vi "Aircraft 8 RC Values .vi"(7 "Method":enum16{"Get", "Set"}(ring), 11 "Aircraft RC Data":T1) -> (3 "Aircraft RC Data 2":T1)   [LabVIEW 2014]
uses:
  Controls/Aircraft RC Data.ctl
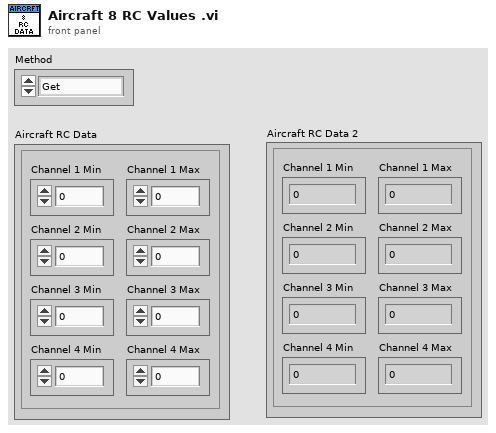
[diagram p1: front panel]
types:
  T1 = typedef "Aircraft RC Data.ctl" = cluster{"Channel 1 Min":i16, "Channel 1 Max":i16, "Channel 2 Min":i16, "Channel 2 Max":i16, "Channel 3 Min":i16, "Channel 3 Max":i16, "Channel 4 Min":i16, "Channel 4 Max":i16}
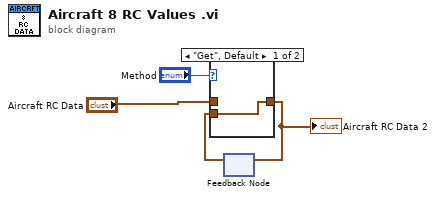
[diagram p0: block diagram]
diagram:
  n1 = feedback #1() -> (w3:T1)  [unwired: 1 in]
  n2 = case shown="\"Get\", Default" "Method" {
    tunnel: "Aircraft RC Data" -> [_ w6]
    tunnel: [w5 w6] -> w2
    tunnel: w3 -> [w5 _]
    frame "Get", Default {
    }
    frame "Set" {
    }
  }
  "Aircraft RC Data 2" <- w2
  n3 = feedback-in #1(w2) -> ()
